vi "Collapsed Terminal Bounds.vi"(9 "Border Without Terminals":T1, 10 "Input":bool, 11 "Index":i32) -> (3 "Bounds":T2)   [LabVIEW 2020, in "Parallel Diagram Block.xnode"]
uses:
  Parallel Diagram Block.xnode
  <vilib>/XNodeSupport/XNodeRect32.ctl
  <vilib>/XNodeSupport/XNodeInt.ctl
  <vilib>/XNodeSupport/NI_XNodeSupport.lvlib
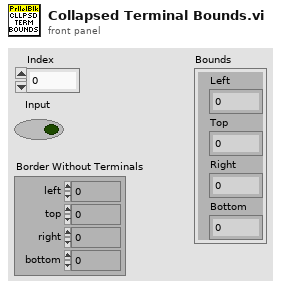
[diagram p1: front panel]
types:
  T1 = cluster{"left":i16, "top":i16, "right":i16, "bottom":i16}
  T2 = typedef "NI_XNodeSupport.lvlib/XNodeRect32.ctl" = cluster{"Left":T3, "Top":T3, "Right":T3, "Bottom":T3}
  T3 = typedef "NI_XNodeSupport.lvlib/XNodeInt.ctl" = i32
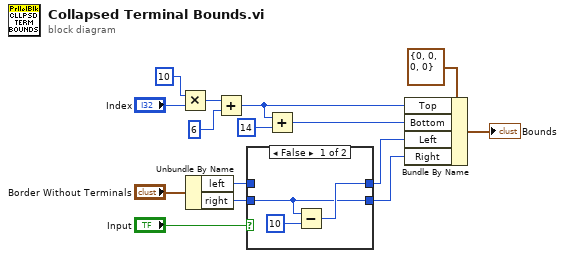
[diagram p0: block diagram]
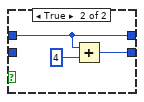
[diagram p2: hidden frame]
diagram:
  n1 = Multiply(x=10 ("y"), y="Index") -> (x*y=w15:i32)
  n2 = Unbundle By Name("Border Without Terminals") -> ("left"=w8:i16, "right"=w9:i16)
  n3 = Add(x=w15, y=6) -> (x+y=w12:i32)
  n4 = case shown="False" "Input" {
    tunnel: w9 -> [w16 _]
    tunnel: w8 -> [_ w19]
    tunnel: [w17 w19] -> w7
    tunnel: [w16 w20] -> w6
    frame False {
      n5 = Subtract(x=w16, y=i16 10) -> (x-y=w17:i16)
    }
    frame True {
      n6 = Add(x=w19, y=i16 4) -> (x+y=w20:i16)
    }
  }
  n7 = Add(x=w12, y=14) -> (x+y=w10:i32)
  n8 = Bundle By Name(cluster=T2 {"Left"=0, "Top"=0, "Right"=0, "Bottom"=0} ("Bounds"), "Top"=w12, "Bottom"=w10, "Left"=w7, "Right"=w6) -> (→"Bounds":T2)
